vi "GetOwningLibrary.vi"(10 "Parent":refnum<vi>) -> (2 "Owner":refnum<vi>)   [LabVIEW 2019]
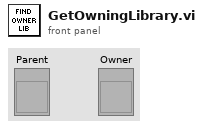
[diagram p1: front panel]
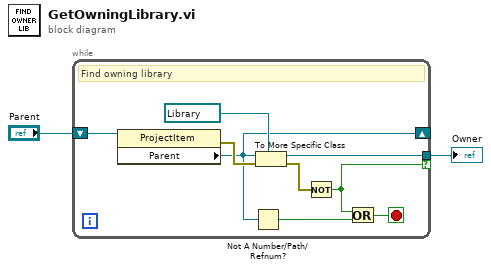
[diagram p0: block diagram]
diagram:
  n1 = while {
    shift-right: [w7] -> _
    shift-left: "Parent" -> [w11]
    tunnel: [w8] -> w1 if=w3
    stop <- w6 stop-if-true
    # "Find owning library"
    n2 = property class="ProjectItem"(reference=w11) -> (error out=w10:errorcluster, "Parent"=w7:refnum<vi>)  [unwired: 1 in, 1 out]
    n3 = Not A Number/Path/Refnum?(number/path/refnum=w7) -> (NaN/Path/Refnum?=w5:bool)
    n4 = To More Specific Class(target class=refnum<vi> refnum ("reference out"), reference=w7, error in=w10) -> (specific class reference=w8:refnum<vi>, error out=w4:errorcluster)
    n5 = Not(x=w4) -> (.not. x?=w3:bool)
    n6 = Or(x=w3, y=w5) -> (x .or. y?=w6:bool)
  }
  "Owner" <- w1
